vi "RunTest - Test Parameter (eFGV).vi"(7 "Action":T5, 8 "error in":errorcluster, 11 "Test Param":T4 {"Data"."Test Type" items=["Please Select", "Triaxial Shear", "Triaxial UU", "Shearbox", "Permeability", "Consolidation (Stepped Loading)/Swelling", "Saturation (Incremental)", "User Defined", "UCT", "Isotropic Consolidation"]}) -> (0 "error out":errorcluster, 2 "Test Param ref":refnum<user-event>, 3 "Test Param out":T4 {"Data"."Test Type" items=["Please Select", "Triaxial Shear", "Triaxial UU", "Shearbox", "Permeability", "Consolidation (Stepped Loading)/Swelling", "Saturation (Incremental)", "User Defined", "UCT", "Isotropic Consolidation"]})   [LabVIEW 2019]
uses:
  Controls/eFGV States.ctl
  Controls/Test Panel - Data Structure.ctl
  Controls/Station - Test Type.ctl
  <vilib>/Utility/miscctls.llb/LVRowAndColumnTypeDef.ctl
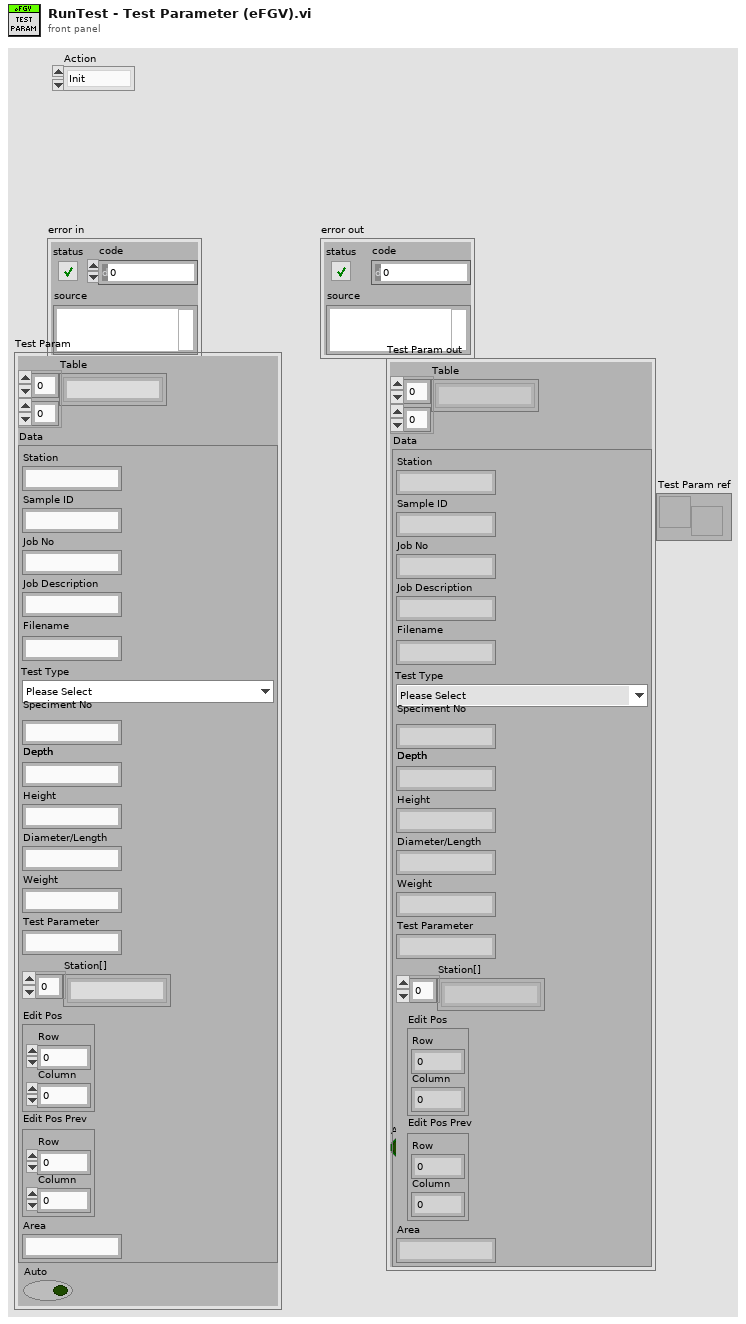
[diagram p1: front panel]
types:
  T1 = typedef "Test Panel - Data Structure.ctl" = cluster{"Station":string, "Sample ID":string, "Job No":string, "Job Description":string, "Filename":string, "Test Type":T2, "Speciment No":string, "Depth":string, "Height":string, "Diameter/Length":string, "Weight":string, "Test Parameter":string, "Station[]":string[], "Edit Pos":T3, "Edit Pos Prev":T3, "Area":string}
  T2 = typedef "Station - Test Type.ctl" = u16
  T3 = typedef "LVRowAndColumnTypeDef.ctl" = cluster{"Row":i32, "Column":i32}
  T4 = cluster{"Table":string[][], "Data":T1, "Auto":bool}
  T5 = typedef "eFGV States.ctl" = enum16{"Init", "Read", "Write", "Exit"}
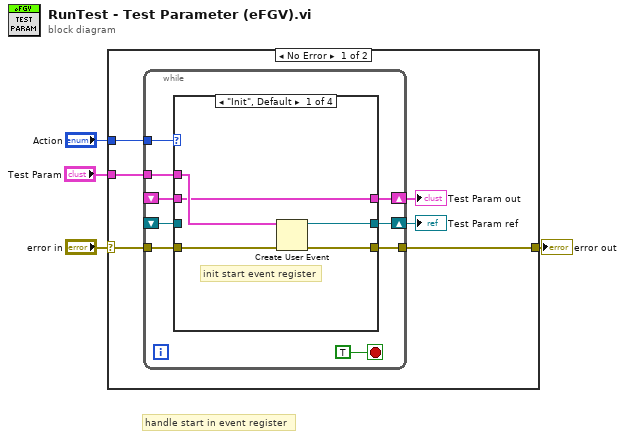
[diagram p0: block diagram]
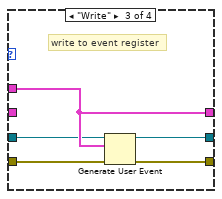
[diagram p3: hidden frame]
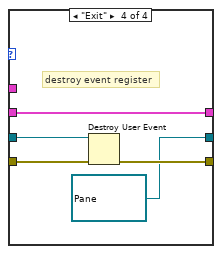
[diagram p4: hidden frame]
diagram:
  # "handle start in event register"
  n1 = case shown="No Error" "error in" {
    selector: "error in" -> [w8 w38]
    tunnel: "Action" -> [w10 _]
    tunnel: "Test Param" -> [w7 _]
    tunnel: [w9 w38] -> w3
    frame No Error {
      n2 = while {
        tunnel: w10 -> [w18]
        tunnel: w8 -> [w16]
        tunnel: [w15] -> w9
        shift-right: [w14] -> w6
        shift-left: _ -> [w17]
        tunnel: w7 -> [w13]
        shift-right: [w12] -> w5
        shift-left: _ -> [w11]
        stop <- TRUE stop-if-true
        n3 = case shown="\"Init\", Default" w18 {
          tunnel: w17 -> [w21 w26 _ w35]
          tunnel: w16 -> [w24 w27 w30 w37]
          tunnel: [w23 w27 w32 w36] -> w15
          tunnel: [w21 w26 w31 w35] -> w14
          tunnel: w13 -> [w22 _ w31 _]
          tunnel: w11 -> [_ w25 w29 w34]
          tunnel: [w20 w25 w28 refnum<user-event> refnum ("Test Param")] -> w12
          frame "Init", Default {
            # "init start event register"
            n4 = Create User Event(user event datatype=w22, error in=w24) -> (user event=w20:refnum<user-event>, error out=w23:errorcluster)
          }
          frame "Read" {
            # "read from event register"
          }
          frame "Write" {
            # "write to event register"
            n5 = Generate User Event(user event=w29, event data cluster=w31, error in=w30) -> (user event out=w28:refnum<user-event>, error out=w32:errorcluster)  [unwired: 1 in]
          }
          frame "Exit" {
            # "destroy event register"
            n6 = Destroy User Event(user event=w34, error in=w37) -> (error out=w36:errorcluster)
          }
        }
      }
      "Test Param out" <- w6
      "Test Param ref" <- w5
    }
    frame Error {
    }
  }
  "error out" <- w3
